vi "Calibration Sample Remove.vi"(8 "error in (no error)":errorcluster, 11 "App in":refnum<class "App.lvclass">) -> (0 "error out":errorcluster, 3 "App out":refnum<class "App.lvclass">)   [LabVIEW 2020, in "AR Example.lvlib" / "App.lvclass"]
uses:
  App.lvclass
  App.lvclass/App.ctl
  UI/UI.lvclass
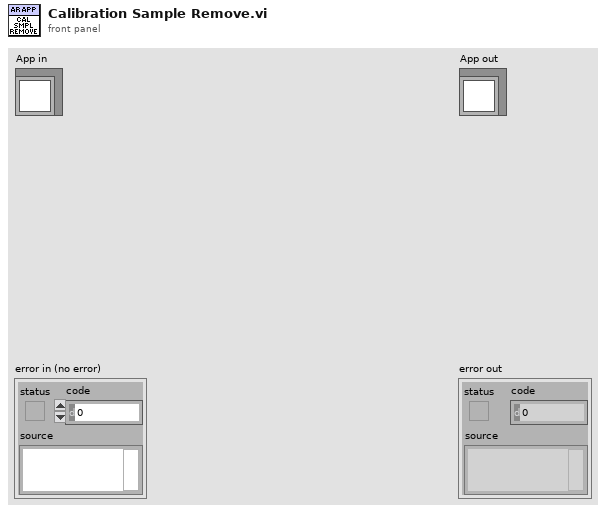
[diagram p1: front panel]
types:
  T1 = typedef "g_ar_toolkit.feature_detection.lvlib/AprilTag Detector.lvclass/Detection.ctl" = cluster{"ID":i32, "Hamming":i32, "Decision Margin":sgl, "Centre":T2, "Corners":T3}
  T2 = typedef "g_ar_toolkit.common.lvlib/Image Point (Float).ctl" = cluster{"x":dbl, "y":dbl}
  T3 = typedef "g_ar_toolkit.common.lvlib/Square Corners.ctl" = cluster{"Bottom Left":T2, "Bottom Right":T2, "Top Right":T2, "Top Left":T2}
  T4 = cluster{"Detections":T1[], "Cal Image":refnum<data-value>}[]
  T5 = cluster{"Detections":T1[], "Cal Image":refnum<data-value>}
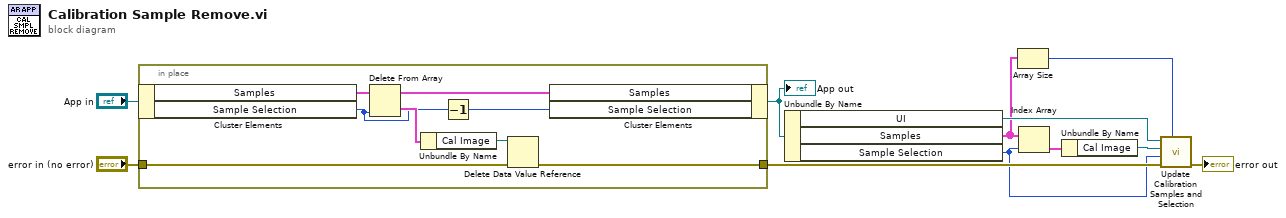
[diagram p0: block diagram]
diagram:
  n1 = in-place {
    in-place-border: "error in (no error)" -> [w14]
    in-place-border: [w15] -> w7
    n2 = in-place-cluster #1("App in") -> ("Samples"=w19:T4, "Sample Selection"=w16:i32)
    n3 = Delete From Array(array=w19, index=w16) -> (deleted portion=w18:T5, array with subset deleted=w13:T4)  [unwired: 1 in]
    n4 = Unbundle By Name(w18) -> ("Cal Image"=w17:refnum<data-value>)
    n5 = Decrement(x=w16) -> (x-1=w12:i32)
    n6 = Delete Data Value Reference(data value reference=w17, error in=w14) -> (error out=w15:errorcluster)  [unwired: 1 out]
    n7 = in-place-cluster #1("Samples"=w13, "Sample Selection"=w12) -> (w9:refnum<class "App.lvclass">)
  }
  "App out" <- w9
  n8 = Unbundle By Name(w9) -> ("UI"=w8:refnum<class "UI.lvclass">, "Samples"=w4:T4, "Sample Selection"=w1:i32)
  n9 = Array Size(array=w4) -> (size(s)=w5:i32)
  n10 = Index Array(array=w4, index=w1) -> (element=w3:T5)
  n11 = Unbundle By Name(w3) -> ("Cal Image"=w2:refnum<data-value>)
  n12 = call "Update Calibration Samples and Selection.vi"("N-Samples"=w5, "error in (no error)"=w7, "Selection"=w1, "Sample"=w2, "UI in"=w8) -> ("error out"=→"error out":errorcluster)  [unwired: 6 in]
